vi "Pre Method Reset.vi"(10 "VI Refnum":refnum<vi>, 11 "LUnit Test Case In":refnum<class "LUnit Test Case.lvclass">) -> (2 "VI Refnum out":refnum<vi>, 3 "LUnit Test Case Out":refnum<class "LUnit Test Case.lvclass">)   [LabVIEW 2020, in "LUnit Test Case.lvclass"]
uses:
  LUnit Test Case.lvclass
  LUnit Test Case.lvclass/LUnit Test Case.ctl
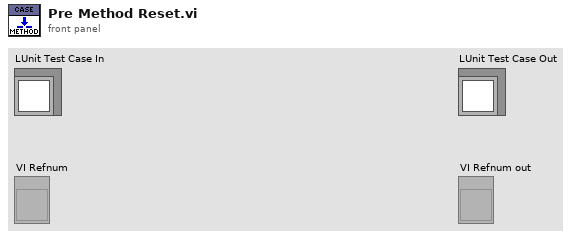
[diagram p1: front panel]
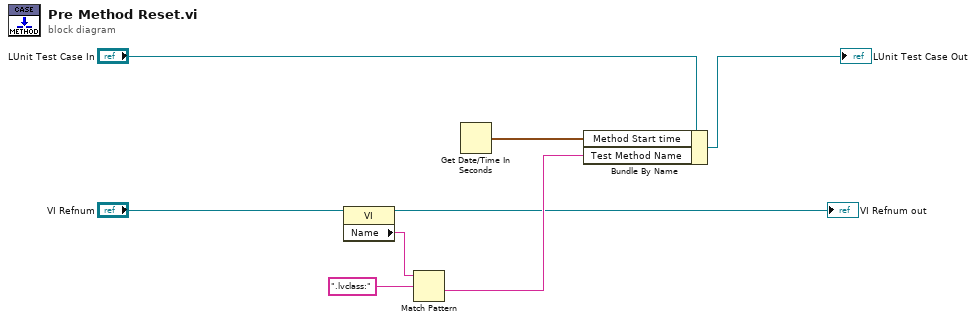
[diagram p0: block diagram]
diagram:
  n1 = property class="VI"(reference="VI Refnum") -> (reference out=→"VI Refnum out":refnum<vi>, "Name"=w4:string)  [unwired: 1 in, 1 out]
  n2 = Match Pattern(string=w4, regular expression=".lvclass:") -> (after substring=w2:string)  [unwired: 1 in, 3 out]
  n3 = Get Date/Time In Seconds() -> (seconds since 1Jan1904=w6:timestamp)
  n4 = Bundle By Name(cluster="LUnit Test Case In", "Method Start time"=w6, "Test Method Name"=w2) -> (→"LUnit Test Case Out":refnum<class "LUnit Test Case.lvclass">)
